vi "Get pin Status Response.vi"(8 "error in (no error)":errorcluster, 11 "Arduino in":refnum<class "Arduino.lvclass">) -> (0 "error out":errorcluster, 2 "Value":string, 3 "Arduino out":refnum<class "Arduino.lvclass">)   [LabVIEW 2020, in "Arduino.lvclass"]
uses:
  Arduino.lvclass
  Abstracts/Serial Device/Serial Device.lvclass
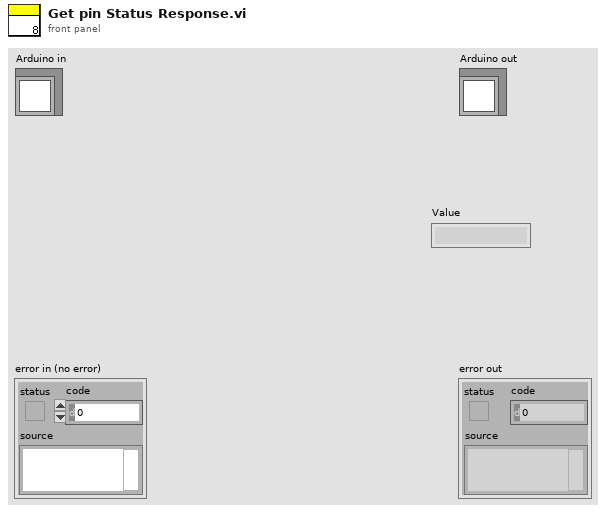
[diagram p1: front panel]
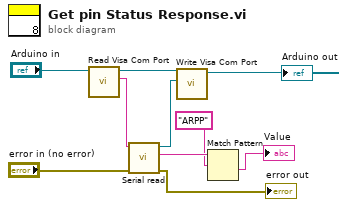
[diagram p0: block diagram]
diagram:
  n1 = call-dynamic "Read Visa Com Port.vi"("Serial Device in"="Arduino in") -> ("Visa Com Port"=w10:string, "Serial Device out"=w6:refnum<class "Arduino.lvclass">)  [unwired: 8 in, 1 out]
  n2 = call "Serial read.vi"("error in (no error)"="error in (no error)", "VISA resource name in"=w10) -> ("error out"=→"error out":errorcluster, "Respuesta"=w4:string, "VISA resource name out"=w9:refnum<visa-resource-name>)  [unwired: 7 in]
  n3 = call-dynamic "Write Visa Com Port.vi"("Visa Com Port"=w9, "Serial Device in"=w6) -> ("Serial Device out"=→"Arduino out":refnum<class "Arduino.lvclass">)  [unwired: 8 in, 1 out]
  n4 = Match Pattern(string=w4, regular expression="ARPP") -> (after substring=→"Value":string)  [unwired: 1 in, 3 out]
